vi "Eat.vi"(8 "error in (no error)":errorcluster, 10 "String":string, 11 "Sheep in":refnum<class "Sheep.lvclass">) -> (0 "error out":errorcluster, 2 "String 2":string, 3 "Sheep out":refnum<class "Sheep.lvclass">)   [LabVIEW 2018, in "Sheep.lvclass"]
uses:
  Sheep.lvclass
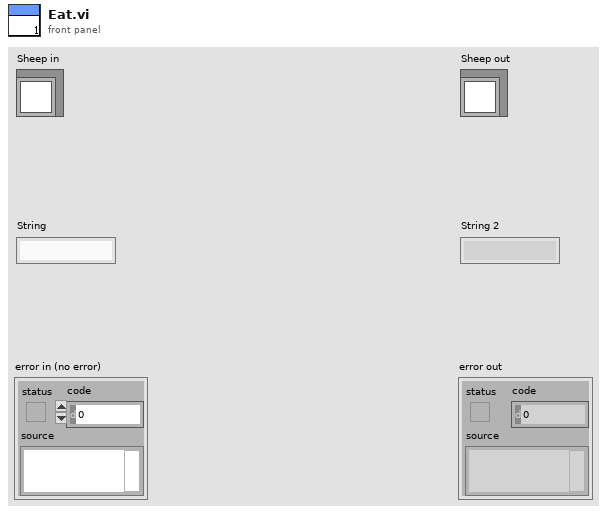
[diagram p1: front panel]
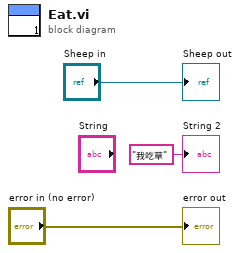
[diagram p0: block diagram]
diagram:
  "error out" <- "error in (no error)"
  "Sheep out" <- "Sheep in"
  "String 2" <- "我吃草" ("String 2")
